vi "To Notification Key.vi"(1 "Alias":string, 4 "Symbol Name":string) -> (6 "Key":string)   [LabVIEW 2018, in "TwinCAT ADS.lvclass"]
uses:
  TwinCAT ADS.lvclass
  Controls/ADS Notification Map Key.ctl
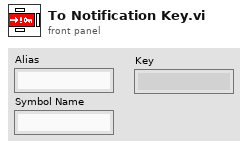
[diagram p1: front panel]
types:
  T1 = typedef "TwinCAT ADS.lvclass/ADS Notification Map Key.ctl" = cluster{"Alias":string, "Symbol Name":string}
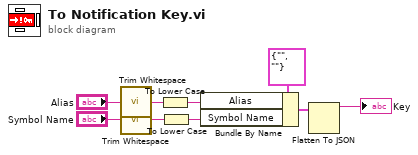
[diagram p0: block diagram]
diagram:
  n1 = call <vilib>:"Trim Whitespace.vi"("string"="Alias") -> ("trimmed string"=w4:string)  [unwired: 1 in]
  n2 = call <vilib>:"Trim Whitespace.vi"("string"="Symbol Name") -> ("trimmed string"=w5:string)  [unwired: 1 in]
  n3 = To Lower Case(string=w4) -> (all lower case string=w2:string)
  n4 = To Lower Case(string=w5) -> (all lower case string=w1:string)
  n5 = Bundle By Name(cluster=T1 {"Alias"="", "Symbol Name"=""} ("Notification User Data"), "Alias"=w2, "Symbol Name"=w1) -> (w9:T1)
  n6 = Flatten To JSON(anything=w9) -> (JSON string=→"Key":string)  [unwired: 2 in, 1 out]
